vi "SetFrictionVoltages.vi"(9 "FricModelParam":T1(array[cluster]), 11 "EncoderVelocity(RPM)":dbl[](array[numeric])) -> (3 "FrictionVoltages":dbl[](array[numeric]))   [LabVIEW 2017]
uses:
  <vilib>/imath/engines/lvmath2/RunTimeEngine/NodeEndStatement/NIMS_NodeEndStatement_Output.vi
  <instcachedir>/0/NIMS_NodeEndStatement_Output_53EC0D466D134D7ABD903AC30B43404B.lvgen/NIMS_NodeEndStatement_Output_53EC0D466D134D7ABD903AC30B43404B_001.vi
  <vilib>/imath/engines/lvmath2/RunTimeEngine/ErrorHandling/NIMS_Finalize Error.vi
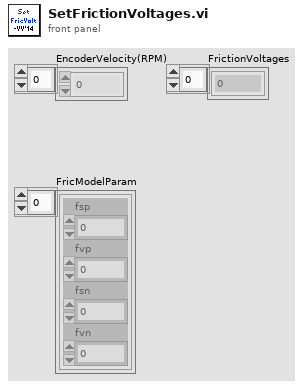
[diagram p1: front panel]
types:
  T1 = cluster{"fsp":dbl, "fvp":dbl, "fsn":dbl, "fvn":dbl}[]
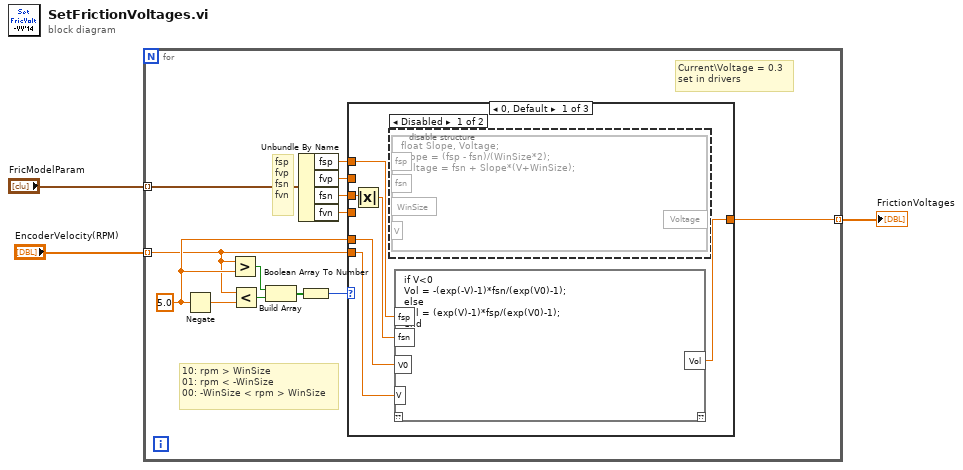
[diagram p0: block diagram]
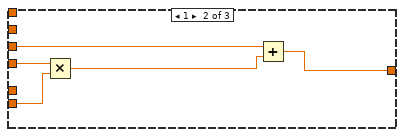
[diagram p3: hidden frame]
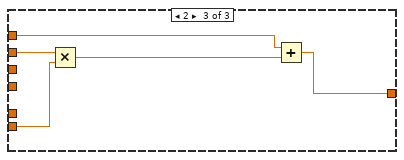
[diagram p4: hidden frame]
diagram:
  n1 = for {
    tunnel: "EncoderVelocity(RPM)" -> [w6] mode=indexing
    tunnel: "FricModelParam" -> [w4] mode=indexing
    tunnel: [w5] -> w3 mode=indexing
    w9 = 5.0 ("y")
    # "10: rpm > WinSize\n01: rpm < -WinSize\n00: -WinSize < rpm > WinSize"
    # "fsp\nfvp\nfsn\nfvn"
    # "Current\\Voltage = 0.3\nset in drivers"
    n2 = Negate(x=w9) -> (-x=w14:dbl)
    n3 = Greater?(x=w6, y=w9) -> (0:w15:bool)
    n4 = Less?(x=w6, y=w14) -> (x < y?=w13:bool)
    n5 = Build Array(w15, w13) -> (w16:bool[])
    n6 = Unbundle By Name(w4) -> ("fsp"=w11:dbl, "fvp"=w7:dbl, "fsn"=w10:dbl, "fvn"=w8:dbl)
    n7 = Boolean Array To Number(Boolean array=w16) -> (number=w12:u32)
    n8 = case shown="0, Default" w12 {
      tunnel: w11 -> [w18 _ w96]
      tunnel: w10 -> [w17 w92 _]
      tunnel: w9 -> [w20 _ _]
      tunnel: w6 -> [w21 w93 w97]
      tunnel: [w19 w90 w95] -> w5
      tunnel: w8 -> [_ w94 _]
      tunnel: w7 -> [_ _ w98]
      frame 0, Default {
        n9 = Absolute Value(x=w17) -> (abs(x)=w22:dbl)
        n10 = disable-structure shown="Disabled" {
          frame Disabled {
            n11 = formula code="float Slope, Voltage;\nSlope = (fsp - fsn)/(WinSize*2);\nVoltage = fsn + Slope*(V+WinSize);"() -> ()  [unwired: 4 in, 1 out]
          }
          frame Enabled {
          }
        }
        n12 = mathscript code="if V<0\nVol = -(exp(-V)-1)*fsn/(exp(V0)-1);\nelse\nVol = (exp(V)-1)*fsp/(exp(V0)-1);\nend"("fsp"=w18, "fsn"=w22, "V"=w21, "V0"=w20) -> ("Vol"=w19:dbl)  [unwired: 1 in, 1 out]
      }
      frame 1 {
        n13 = Multiply(x=w94, y=w93) -> (x*y=w91:dbl)
        n14 = Add(x=w92, y=w91) -> (x+y=w90:dbl)
      }
      frame 2 {
        n15 = Multiply(x=w98, y=w97) -> (x*y=w99:dbl)
        n16 = Add(x=w96, y=w99) -> (x+y=w95:dbl)
      }
    }
  }
  "FrictionVoltages" <- w3
